vi "Test Serialize Void.vi"(8 "error in (no error)":errorcluster) -> (0 "error out":errorcluster)   [LabVIEW 2013]
uses:
  src/Serializer/JSON Serializer/JSON Serializer.lvclass
  <vilib>/addons/_JKI Toolkits/Caraya/classes/Test/Test.lvclass
  <vilib>/addons/_JKI Toolkits/Caraya/classes/Assert/Assert.lvclass
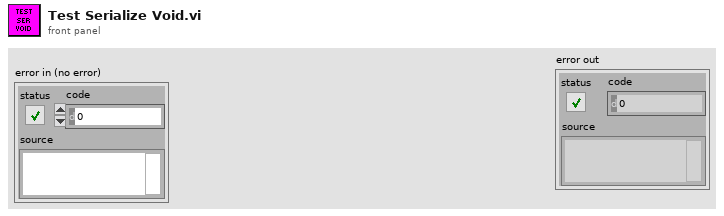
[diagram p1: front panel]
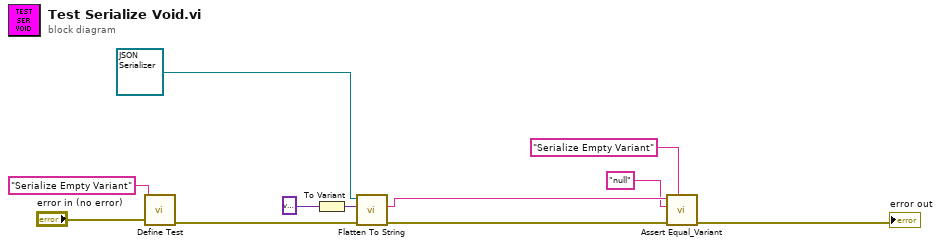
[diagram p0: block diagram]
diagram:
  n1 = call <vilib>:"Define Test.vi"("error in (no error)"="error in (no error)", "Label (VI Title)"="Serialize Empty Variant") -> ("error out"=w8:errorcluster)  [unwired: 9 in]
  n2 = To Variant(anything=variant) -> (Variant=w2:variant)
  n3 = call-dynamic "Flatten To String.vi"("error in (no error)"=w8, "Variant"=w2, "JSON Serializer in"=refnum<class "JSON Serializer.lvclass"> refnum ("JKI JSON Serialization.lvlib:JSON Serializer.lvclass")) -> ("error out"=w7:errorcluster, "String"=w5:string)  [unwired: 6 in, 1 out]
  n4 = call <vilib>:"Assert Equal_Variant.vi"("Label"="Serialize Empty Variant", "error in (no error)"=w7, "Y"="null", "X"=w5) -> ("error out"=→"error out":errorcluster)  [unwired: 7 in]
